vi "Get Compiled Counter And Protection Incoming Frames.vi"(0 "XNET Cluster":refnum<k21>, 5 "GUIDs":T11, 7 "Incoming Frames In":T2 {"Frame Settings"."Tx Control.Override Period Value Ref" format="%.0x"; "Frame Settings"."Tx Control.Override Period Ref" format="%.0x"; "Frame Settings"."Tx Control.Disable Tx Ref" format="%.0x"; "Frame Settings"."Transmit Trigger Ref" format="%.0x"; "Frame Settings"."Disable Transmission Ref" format="%.0x"; "Frame Refs" format="%.0x"}, 11 "error in (no error)":errorcluster) -> (4 "Incoming Frames Out":T6[](array[typedef]) {"Protection Configurations"."CRC Channels"."Data Type" items=["Signed", "Unsigned", "IEEE Float"]}, 6 "Signals Refs":T1[](array[typedef]) format="%.0x", 8 "Counters and Protection Refs":T1[](array[typedef]) format="%.0x", 10 "Invalid Refs":T1[](array[typedef]) format="%.0x", 13 "Rcv Time Refs":T1[](array[typedef]) format="%.0x", 14 "Time Diff Refs":T1[](array[typedef]) format="%.0x", 15 "error out":errorcluster)   [LabVIEW 2023, in "Protection and Counter Support System Explorer.lvlib"]
uses:
  Protection and Counter Support System Explorer.lvlib
  Types/Export Frame GUIDs List.ctl
  Shared/Types/Exported Frame Settings.ctl
  Shared/Types/Exported Frame Type.ctl
  Shared/Types/Exported Protection Settings.ctl
  Shared/Types/Protection Type.ctl
  Shared/Types/XNET Signal Configuration.ctl
  Shared/Types/Exported Counter Settings.ctl
  Shared/Types/Exported Event Trigger Type.ctl
  <vilib>/NI VeriStand/Custom Device API/Custom Device Item Ref.ctl
  Types/Export Frames List and Type.ctl
  Types/Exported Frame Settings.ctl
  <vilib>/NI VeriStand/Custom Device Tools/Custom Device Utility Library/NI VeriStand - Search for All Items by GUID.vi
  <vilib>/NI VeriStand/Custom Device Tools/Custom Device Utility Library/NI VeriStand - Search for Item by GUID.vi
  Shared/Protection and Counter Support Shared.lvlib
  <vilib>/NI VeriStand/Custom Device API/Custom Device API.lvlib
  <resource>/objmgr/xnet.rc
  <vilib>/NI VeriStand/Custom Device Tools/Custom Device Utility Library/Custom Device Utility Library.lvlib
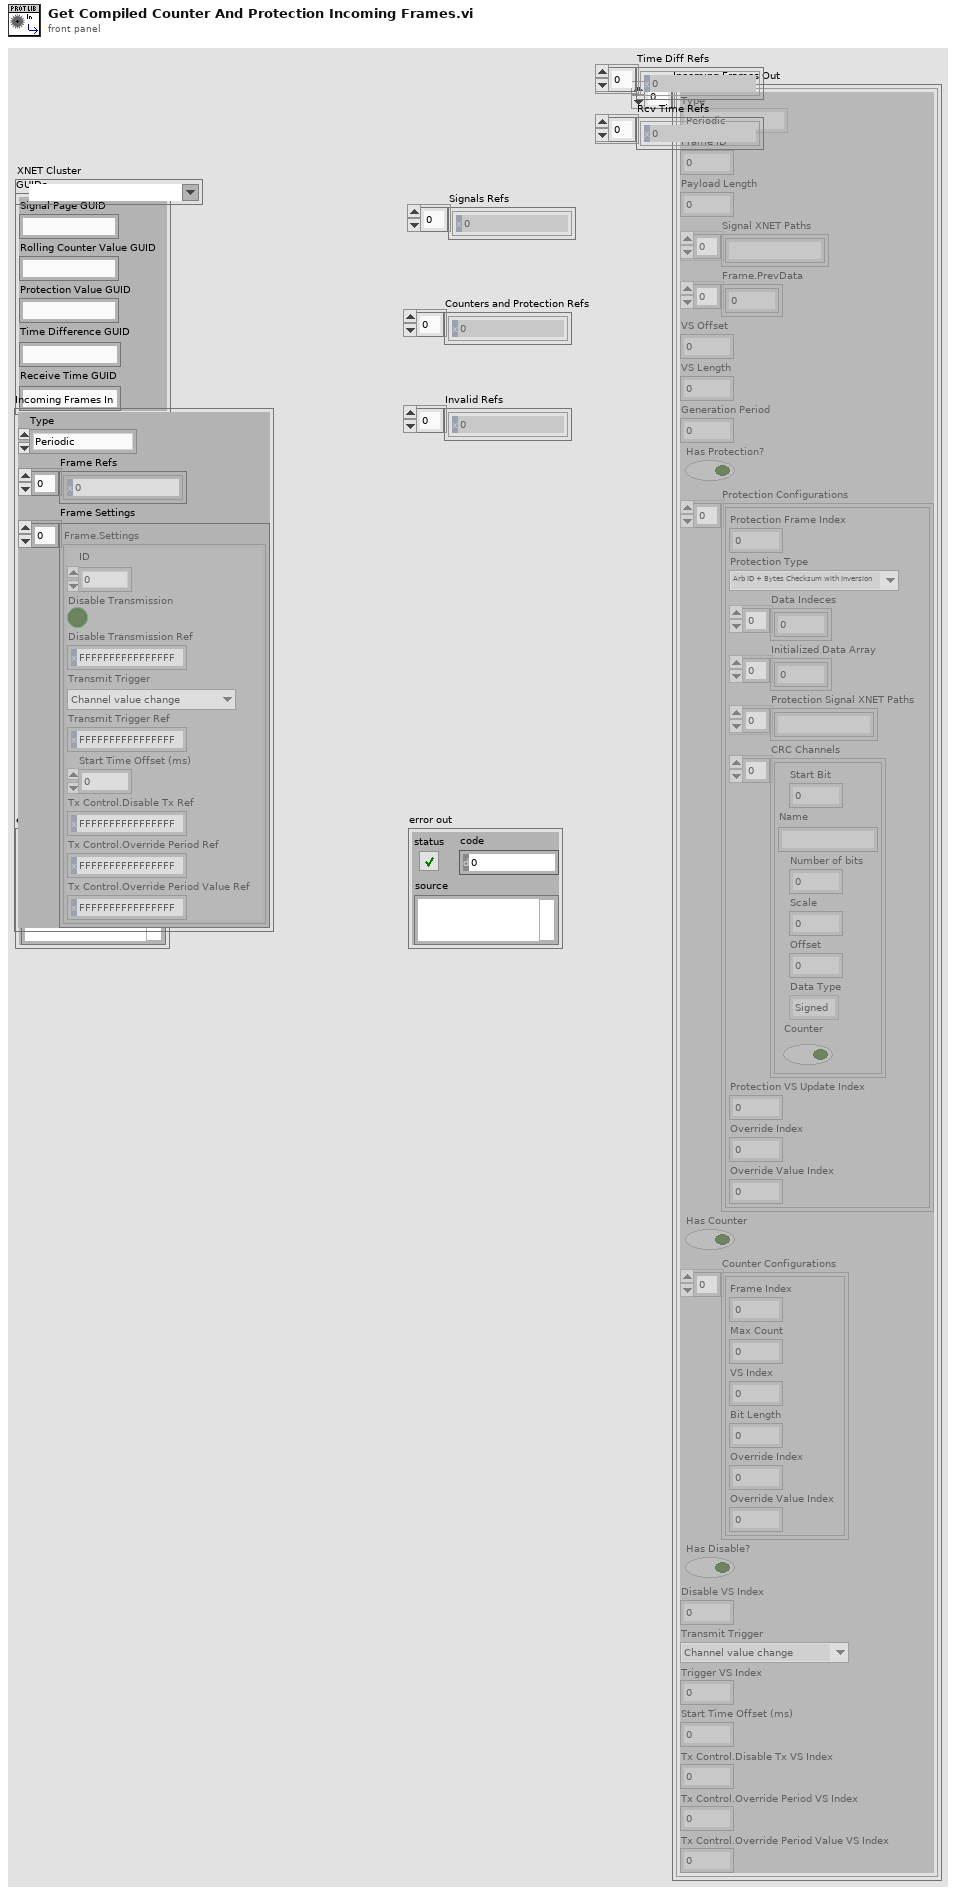
[diagram p1: front panel]
types:
  T1 = typedef "Custom Device API.lvlib/Custom Device Item Ref.ctl" = u64
  T2 = typedef "Protection and Counter Support System Explorer.lvlib/Export Frames List and Type.ctl" = cluster{"Type":T3, "Frame Refs":T1[], "Frame Settings":T4[]}
  T3 = typedef "Protection and Counter Support Shared.lvlib/Exported Frame Type.ctl" = enum16{"Periodic", "Event", "Periodic/Event"}
  T4 = typedef "Protection and Counter Support System Explorer.lvlib/Exported Frame Settings.ctl" = cluster{"ID":u32, "Disable Transmission":bool, "Disable Transmission Ref":T1, "Transmit Trigger":T5, "Transmit Trigger Ref":T1, "Start Time Offset (ms)":u32, "Tx Control.Disable Tx Ref":T1, "Tx Control.Override Period Ref":T1, "Tx Control.Override Period Value Ref":T1}
  T5 = typedef "Protection and Counter Support Shared.lvlib/Exported Event Trigger Type.ctl" = enum16{"Channel value change", "Trigger channel (not zero)", "Channel value change or trigger channel (not zero)", "Trigger channel (any value change)", "Channel value change or trigger channel (any value change)"}
  T6 = typedef "Protection and Counter Support Shared.lvlib/Exported Frame Settings.ctl" = cluster{"Type":T3, "Frame ID":u32, "Payload Length":u32, "Signal XNET Paths":string[], "Frame.PrevData":dbl[], "VS Offset":i32, "VS Length":i32, "Generation Period":u32, "Has Protection?":bool, "Protection Configurations":T7[], "Has Counter":bool, "Counter Configurations":T10[], "Has Disable?":bool, "Disable VS Index":i32, "Transmit Trigger":T5, "Trigger VS Index":i32, "Start Time Offset (ms)":u32, "Tx Control.Disable Tx VS Index":i32, "Tx Control.Override Period VS Index":i32, "Tx Control.Override Period Value VS Index":i32}
  T7 = typedef "Protection and Counter Support Shared.lvlib/Exported Protection Settings.ctl" = cluster{"Protection Frame Index":i32, "Protection Type":T8, "Data Indeces":i32[], "Initialized Data Array":dbl[], "Protection Signal XNET Paths":string[], "CRC Channels":T9[], "Protection VS Update Index":i32, "Override Index":i32, "Override Value Index":i32}
  T8 = typedef "Protection and Counter Support Shared.lvlib/Protection Type.ctl" = enum16{"Arb ID + Bytes Checksum with Inversion", "Arb ID + Bytes CRC with Inversion", "Reversed Raw Signal Checksum with Inversion", "Concatenated Two's Compliment", "LP_CRC8", "LP_Checksum", "LP_CRC8_MRS"}
  T9 = typedef "Protection and Counter Support Shared.lvlib/XNET Signal Configuration.ctl" = cluster{"Start Bit":i32, "Name":string, "Number of bits":i32, "Scale":dbl, "Offset":dbl, "Data Type":u32, "Counter":bool}
  T10 = typedef "Protection and Counter Support Shared.lvlib/Exported Counter Settings.ctl" = cluster{"Frame Index":i32, "Max Count":dbl, "VS Index":i32, "Bit Length":i64, "Override Index":i32, "Override Value Index":i32}
  T11 = typedef "Protection and Counter Support System Explorer.lvlib/Export Frame GUIDs List.ctl" = cluster{"Signal Page GUID":string, "Rolling Counter Value GUID":string, "Protection Value GUID":string, "Time Difference GUID":string, "Receive Time GUID":string}
  T12 = typedef "Custom Device API.lvlib/Custom Device Item Info.ctl" = cluster{"Name":string, "Is Channel":bool, "GUID":string, "Is Waveform":bool}
  T13 = typedef "Protection and Counter Support System Explorer.lvlib/Protection Signal Settings.ctl" = cluster{"Input Channels":T14[], "Protection Type":T8}
  T14 = typedef "Protection and Counter Support System Explorer.lvlib/Protection Signal Linked Channel.ctl" = cluster{"Node Ref":T1}
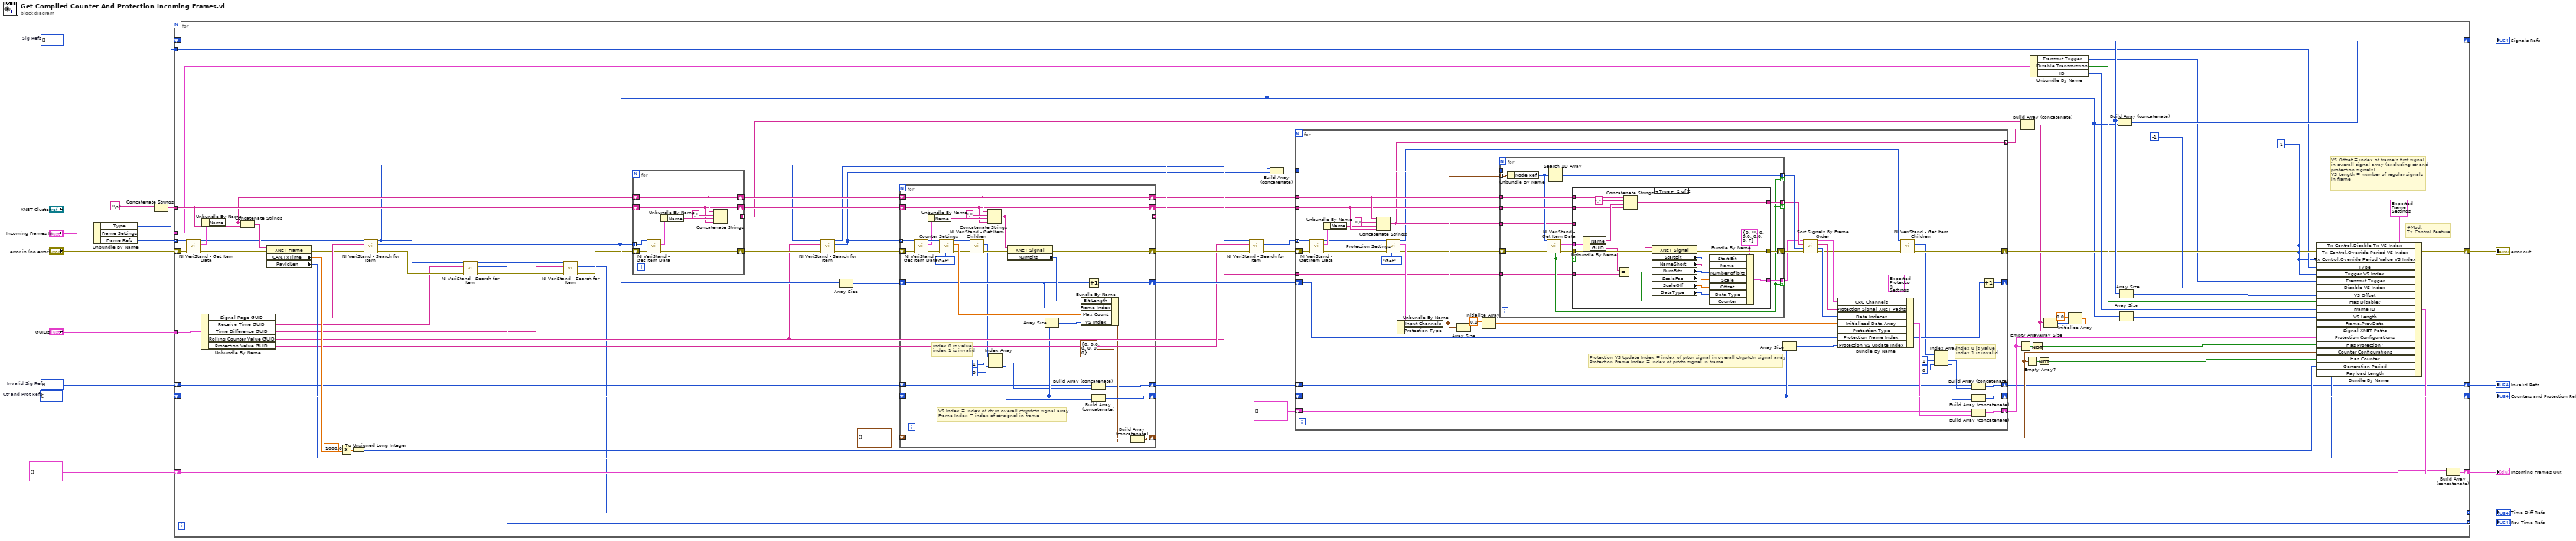
[diagram p0: block diagram]
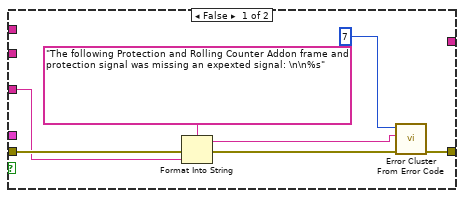
[diagram p2: hidden frame]
diagram:
  w12 = T1[] []  # Invalid Sig Refs
  w18 = T1[] []  # Ctr and Prot Refs
  w17 = T1[] []  # Sig Refs
  n1 = Unbundle By Name("Incoming Frames In") -> ("Type"=w7:T3, "Frame Settings"=w5:T4[], "Frame Refs"=w6:T1[])
  n2 = Concatenate Strings("\n", "XNET Cluster") -> (w8:string)
  n3 = for {
    tunnel: w6 -> [w85] mode=indexing
    shift-right: [w56] -> w10
    shift-left: "error in (no error)" -> [w86]
    shift-right: [w96] -> w1
    shift-left: w17 -> [w95]
    tunnel: w8 -> [w72]
    shift-right: [w50] -> w14
    shift-left: w18 -> [w76]
    shift-right: [w43] -> w15
    shift-left: T6[] [] -> [w42]
    tunnel: w7 -> [w41]
    tunnel: "GUIDs" -> [w40]
    tunnel: w5 -> [w37] mode=indexing
    shift-right: [w31] -> w11
    shift-left: w12 -> [w33]
    tunnel: [w25] -> w2 mode=indexing
    tunnel: [w24] -> w3 mode=indexing
    w21 = -1
    # "#Mod:\nTx Control Feature"
    # "VS Offset = index of frame's first signal\nin overall signal array (excluding ctr and\nprotection signals)\nVS Length = number of regular signals\nin frame"
    n4 = call <vilib>:"NI VeriStand - Get Item Data.vi"("error in (no error)"=w86, "Item Ref in"=w85) -> ("error out"=w82:errorcluster, "Item Info"=w84:T12, "Item Ref out"=w35:T1)  [unwired: 6 in, 1 out]
    n5 = Unbundle By Name(w40) -> ("Signal Page GUID"=w39:string, "Receive Time GUID"=w23:string, "Time Difference GUID"=w22:string, "Rolling Counter Value GUID"=w34:string, "Protection Value GUID"=w38:string)
    n6 = Unbundle By Name(w84) -> ("Name"=w71:string)
    n7 = Concatenate Strings(w71, w72) -> (w83:string)
    n8 = property class="XNET Frame"(reference=w83, error in=w82) -> (error out=w36:errorcluster, "CAN.TxTime"=w80:dbl, "PayldLen"=w46:u32)  [unwired: 1 out]
    n9 = Multiply(x=1000.0 ("y"), y=w80) -> (x*y=w81:dbl)
    n10 = To Unsigned Long Integer(number=w81) -> (unsigned 32bit integer=w78:u32)
    n11 = call-poly <vilib>:"NI VeriStand - Search for Item.vi"("error in"=w36, "Item GUID"=w39, "Section Ref in"=w35) -> ("error out"=w27:errorcluster, "Item Refs"=w48:T1[], "Section Ref out"=w29:T1)  [unwired: 5 in, 1 out]
    n12 = call-poly <vilib>:"NI VeriStand - Search for Item.vi"("error in"=w27, "Item GUID"=w23, "Section Ref in"=w29) -> ("error out"=w30:errorcluster, "Item Ref"=w25:T1, "Section Ref out"=w28:T1)  [unwired: 5 in, 1 out]
    n13 = call-poly <vilib>:"NI VeriStand - Search for Item.vi"("error in"=w30, "Item GUID"=w22, "Section Ref in"=w28) -> ("error out"=w26:errorcluster, "Item Ref"=w24:T1)  [unwired: 5 in, 2 out]
    n14 = for {
      tunnel: w48 -> [w195] mode=indexing
      shift-right: [w189] -> w73
      shift-left: w26 -> [w194]
      tunnel: [w191] -> w68 mode=indexing
      shift-right: [w188] -> w70
      shift-left: w71 -> [w188]
      shift-right: [w187] -> w69
      shift-left: w72 -> [w187]
      n15 = call <vilib>:"NI VeriStand - Get Item Data.vi"("error in (no error)"=w194, "Item Ref in"=w195) -> ("error out"=w189:errorcluster, "Item Info"=w190:T12)  [unwired: 6 in, 2 out]
      n16 = Unbundle By Name(w190) -> ("Name"=w192:string)
      n17 = Concatenate Strings(w188, "." ("string"), w192, w187) -> (w191:string)
    }
    n18 = call-poly <vilib>:"NI VeriStand - Search for Item.vi"("error in"=w73, "Item GUID"=w34, "Section Ref in"=w29) -> ("error out"=w75:errorcluster, "Item Refs"=w47:T1[], "Section Ref out"=w65:T1)  [unwired: 5 in, 1 out]
    n19 = Array Size(array=w48) -> (size(s)=w74:i32)
    n20 = for {
      tunnel: w47 -> [w228] mode=indexing
      shift-right: [w209] -> w66
      shift-left: w75 -> [w227]
      shift-right: [w224] -> w87
      shift-left: T10[] [] -> [w223]
      tunnel: [w208] -> w67 mode=indexing
      shift-right: [w218] -> w51
      shift-left: w76 -> [w219]
      shift-right: [w213] -> w61
      shift-left: w74 -> [w206]
      shift-right: [w212] -> w59
      shift-left: w70 -> [w212]
      shift-right: [w211] -> w60
      shift-left: w69 -> [w211]
      shift-right: [w202] -> w32
      shift-left: w33 -> [w205]
      # "VS Index = index of ctr in overall ctr/prtctn signal array\nFrame Index = index of ctr signal in frame"
      # "index 0 is value\nindex 1 is invalid"
      n21 = call <vilib>:"NI VeriStand - Get Item Data.vi"("error in (no error)"=w227, "Item Ref in"=w228) -> ("error out"=w225:errorcluster, "Item Info"=w220:T12, "Item Ref out"=w226:T1)  [unwired: 6 in, 1 out]
      n22 = Unbundle By Name(w220) -> ("Name"=w221:string)
      n23 = call "Counter Settings.vi"("Action"=enum8{"Get", "Set"}."Get", "error in"=w225, "Parent Ref"=w226) -> ("error out"=w204:errorcluster, "Max Count"=w217:dbl, "Parent Ref Out"=w200:T1)  [unwired: 6 in]
      n24 = call <vilib>:"NI VeriStand - Get Item Children.vi"("error in (no error)"=w204, "Item Ref in"=w200) -> ("error out"=w203:errorcluster, "Child Refs"=w199:T1[])  [unwired: 6 in, 2 out]
      n25 = Concatenate Strings(w212, "." ("string"), w221, w211) -> (w208:string)
      n26 = Index Array(array=w199, index #1=1 ("length"), index #2=0 ("index")) -> (element #1=w197:T1, element #2=w196:T1)
      n27 = property class="XNET Signal"(reference=w208, error in=w203) -> (error out=w209:errorcluster, "NumBits"=w207:u32)  [unwired: 1 out]
      n28 = Array Size(array=w219) -> (size(s)=w214:i32)
      n29 = Bundle By Name(cluster=T10 {"Frame Index"=0, "Max Count"=0.0, "VS Index"=0, "Bit Length"=0, "Override Index"=0, "Override Value Index"=0} ("Cluster"), "Bit Length"=w207, "Frame Index"=w206, "Max Count"=w217, "VS Index"=w214) -> (w216:T10)
      n30 = Increment(x=w206) -> (x+1=w213:i32)
      n31 = Build Array (concatenate)(w205, w197) -> (w202:T1[])
      n32 = Build Array (concatenate)(w219, w196) -> (w218:T1[])
      n33 = Build Array (concatenate)(w223, w216) -> (w224:T10[])
    }
    n34 = call-poly <vilib>:"NI VeriStand - Search for Item.vi"("error in"=w66, "Item GUID"=w38, "Section Ref in"=w65) -> ("error out"=w64:errorcluster, "Item Refs"=w63:T1[])  [unwired: 5 in, 2 out]
    n35 = Build Array (concatenate)(w48, w47) -> (w49:T1[])
    n36 = for {
      tunnel: w63 -> [w145] mode=indexing
      shift-right: [w106] -> w56
      shift-left: w64 -> [w144]
      shift-right: [w141] -> w57
      shift-left: T7[] [] -> [w143]
      tunnel: w49 -> [w142]
      tunnel: w59 -> [w139]
      tunnel: [w121] -> w58 mode=indexing
      shift-right: [w135] -> w50
      shift-left: w51 -> [w136]
      shift-right: [w123] -> _
      shift-left: w61 -> [w124]
      tunnel: w60 -> [w138]
      tunnel: w34 -> [w119]
      shift-right: [w111] -> w31
      shift-left: w32 -> [w110]
      # "Protection VS Update Index = index of prtcn signal in overall ctr/prtctn signal array\nProtection Frame Index = index of prtctn signal in frame"
      # "index 0 is value\nindex 1 is invalid"
      n37 = call <vilib>:"NI VeriStand - Get Item Data.vi"("error in (no error)"=w144, "Item Ref in"=w145) -> ("error out"=w109:errorcluster, "Item Info"=w137:T12, "Item Ref out"=w108:T1)  [unwired: 6 in, 1 out]
      n38 = Unbundle By Name(w137) -> ("Name"=w122:string)
      n39 = Concatenate Strings(w139, "." ("string"), w122, w138) -> (w121:string)
      n40 = call "Protection Settings.vi"("Action"=enum8{"Get", "Set"}."Get", "error in"=w109, "Parent Ref"=w108) -> ("error out"=w127:errorcluster, "Selected Channels"=w134:T13, "Parent Ref Out"=w105:T1)  [unwired: 6 in]
      n41 = Unbundle By Name(w134) -> ("Input Channels"=w132:T14[], "Protection Type"=w133:T8)
      n42 = Array Size(array=w132) -> (size(s)=w131:i32)
      n43 = Initialize Array(0.0 ("element"), w131) -> (w129:dbl[])
      n44 = for {
        tunnel: w142 -> [w150]
        tunnel: w132 -> [w160] mode=indexing
        tunnel: [w159] -> w118 mode=indexing if=w148
        shift-right: [w153] -> w116
        shift-left: w127 -> [w158]
        tunnel: w139 -> [w156]
        tunnel: w138 -> [w155]
        tunnel: [w151] -> w115 mode=indexing if=w148
        tunnel: [w152] -> w114 mode=indexing if=w148
        tunnel: w121 -> [w147]
        tunnel: w119 -> [w146]
        n45 = Unbundle By Name(w160) -> ("Node Ref"=w149:T1)
        n46 = call <vilib>:"NI VeriStand - Get Item Data.vi"("error in (no error)"=w158, "Item Ref in"=w149) -> ("error out"=w154:errorcluster, "Item Info"=w157:T12, "Found"=w148:bool)  [unwired: 6 in, 1 out]
        n47 = Search 1D Array(1D array=w150, element=w149) -> (index of element=w159:i32)  [unwired: 1 in]
        n48 = case shown="True" w148 {
          tunnel: w157 -> [_ w186]
          tunnel: w156 -> [_ w183]
          tunnel: w155 -> [_ w182]
          tunnel: w154 -> [w165 w181]
          tunnel: [w167 w180] -> w153
          tunnel: [_ w172] -> w152
          tunnel: [_ w171] -> w151
          tunnel: w147 -> [w162 _]
          tunnel: w146 -> [_ w170]
          frame False {
            n49 = Format Into String(format string="The following Protection and Rolling Counter Addon frame and protection signal was missing an expexted signal: \n\n%s" ("error message (\"\")"), error in=w165, w162) -> (resulting string=w161:string, error out=w164:errorcluster)  [unwired: 1 in]
            n50 = call <vilib>:"Error Cluster From Error Code.vi"("error in (no error)"=w164, "error message (\"\")"=w161, "error code (0)"=7) -> ("error out"=w167:errorcluster)  [unwired: 6 in]
          }
          frame True {
            n51 = Unbundle By Name(w186) -> ("Name"=w184:string, "GUID"=w168:string)
            n52 = Equal?(x=w168, y=w170) -> (x = y?=w169:bool)
            n53 = Concatenate Strings(w183, "." ("string"), w184, w182) -> (w171:string)
            n54 = property class="XNET Signal"(reference=w171, error in=w181) -> (error out=w180:errorcluster, "StartBit"=w173:u32, "NameShort"=w174:string, "NumBits"=w175:u32, "ScaleFac"=w176:dbl, "ScaleOff"=w177:dbl, "DataType"=w178:u32)  [unwired: 1 out]
            n55 = Bundle By Name(cluster=T9 {"Start Bit"=0, "Name"="", "Number of bits"=0, "Scale"=0.0, "Offset"=0.0, "Data Type"=0, "Counter"=FALSE} ("MonitoredChannelSettings"), "Start Bit"=w173, "Name"=w174, "Number of bits"=w175, "Scale"=w176, "Offset"=w177, "Data Type"=w178, "Counter"=w169) -> (w172:T9)
          }
        }
      }
      n56 = Array Size(array=w136) -> (size(s)=w125:i32)
      n57 = call "Sort Signals By Frame Order.vi"("error in (no error)"=w116, "Node Refs"=w118, "XNET Paths"=w115, "Signals"=w114) -> ("error out"=w107:errorcluster, "Ordered Node Refs"=w117:i32[], "Ordered XNET Paths"=w112:string[], "Ordered Signals"=w113:T9[])  [unwired: 4 in]
      n58 = Bundle By Name(cluster=T7 {"Protection Frame Index"=0, "Protection Type"=enum."Arb ID + Bytes Checksum with Inversion", "Data Indeces"=[], "Initialized Data Array"=[], "Protection Signal XNET Paths"=[], "CRC Channels"=[], "Protection VS Update Index"=0, "Override Index"=0, "Override Value Index"=0} ("Cluster"), "CRC Channels"=w113, "Protection Signal XNET Paths"=w112, "Data Indeces"=w117, "Initialized Data Array"=w129, "Protection Type"=w133, "Protection Frame Index"=w124, "Protection VS Update Index"=w125) -> (w128:T7)
      n59 = call <vilib>:"NI VeriStand - Get Item Children.vi"("error in (no error)"=w107, "Item Ref in"=w105) -> ("error out"=w106:errorcluster, "Child Refs"=w103:T1[])  [unwired: 6 in, 2 out]
      n60 = Index Array(array=w103, index #1=1 ("length"), index #2=0 ("index")) -> (element #1=w101:T1, element #2=w100:T1)
      n61 = Build Array (concatenate)(w110, w101) -> (w111:T1[])
      n62 = Build Array (concatenate)(w136, w100) -> (w135:T1[])
      n63 = Build Array (concatenate)(w143, w128) -> (w141:T7[])
      n64 = Increment(x=w124) -> (x+1=w123:i32)
    }
    n65 = Empty Array?(array=w57) -> (empty?=w89:bool)
    n66 = Build Array (concatenate)(w68, w67, w58) -> (w55:string[])
    n67 = Empty Array?(array=w87) -> (empty?=w91:bool)
    n68 = Unbundle By Name(w37) -> ("Transmit Trigger"=w45:T5, "Disable Transmission"=w97:bool, "ID"=w98:u32)
    n69 = Not(x=w89) -> (.not. x?=w88:bool)
    n70 = Not(x=w91) -> (.not. x?=w90:bool)
    n71 = Array Size(array=w55) -> (size(s)=w53:i32)
    n72 = Initialize Array(0.0 ("element"), w53) -> (w52:dbl[])
    n73 = Build Array (concatenate)(w95, w48) -> (w96:T1[])
    n74 = Array Size(array=w95) -> (size(s)=w94:i32)
    n75 = Array Size(array=w48) -> (size(s)=w77:i32)
    n76 = Bundle By Name(cluster=T6 {"Type"=enum."Periodic", "Frame ID"=0, "Payload Length"=0, "Signal XNET Paths"=[], "Frame.PrevData"=[], "VS Offset"=0, "VS Length"=0, "Generation Period"=0, "Has Protection?"=FALSE, "Protection Configurations"=[], "Has Counter"=FALSE, "Counter Configurations"=[], "Has Disable?"=FALSE, "Disable VS Index"=0, "Transmit Trigger"=enum."Channel value change", "Trigger VS Index"=0, "Start Time Offset (ms)"=0, "Tx Control.Disable Tx VS Index"=0, "Tx Control.Override Period VS Index"=0, "Tx Control.Override Period Value VS Index"=0} ("Frame Settings"), "Tx Control.Disable Tx VS Index"=w21, "Tx Control.Override Period VS Index"=w21, "Tx Control.Override Period Value VS Index"=w21, "Type"=w41, "Trigger VS Index"=w21, "Transmit Trigger"=w45, "Disable VS Index"=-1, "VS Offset"=w94, "Has Disable?"=w97, "Frame ID"=w98, "VS Length"=w77, "Frame.PrevData"=w52, "Signal XNET Paths"=w55, "Protection Configurations"=w57, "Has Protection?"=w88, "Counter Configurations"=w87, "Has Counter"=w90, "Generation Period"=w78, "Payload Length"=w46) -> (w44:T6)
    n77 = Build Array (concatenate)(w42, w44) -> (w43:T6[])
  }
  "Incoming Frames Out" <- w15
  "error out" <- w10
  "Counters and Protection Refs" <- w14
  "Signals Refs" <- w1
  "Invalid Refs" <- w11
  "Time Diff Refs" <- w3
  "Rcv Time Refs" <- w2
